vi "DatabaseHand_Element_Get(single).vi"(7 "nd queue":bool, 8 "error in (no error)":errorcluster, 9 "default value":sgl format="%.2f", 10 "name":string, 11 "Database RefNum in":T1) -> (0 "error out":errorcluster, 1 "type":string, 2 "value":sgl format="%.2f", 3 "Database RefNum out":T1, 4 "permissions":string="RW", 5 "group":string, 6 "unit":string)   [LabVIEW 2016]
doc: "This VI finds the RefNum of an existing object with the input Name or creates a new object if the Name is not found or Name is unwired or an empty string.\nCopyright 2001 VI Engineering, Inc."
uses:
  DatabaseHand_RefNum.ctl
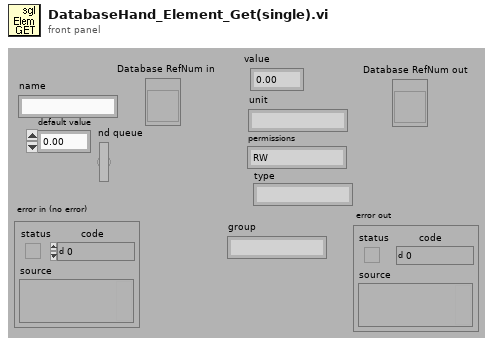
[diagram p1: front panel]
types:
  T1 = typedef "DatabaseHand_RefNum.ctl" = refnum<vi>
  T2 = typedef "DatabaseHand_Element.ctl" = cluster{"name":string, "Database":T3[]}
  T3 = typedef "DatabaseHan_DatabaseElement.ctl" = cluster{"name":string, "value":string, "type":string, "unit":string, "permissions":string, "enqueued":bool, "group":string}
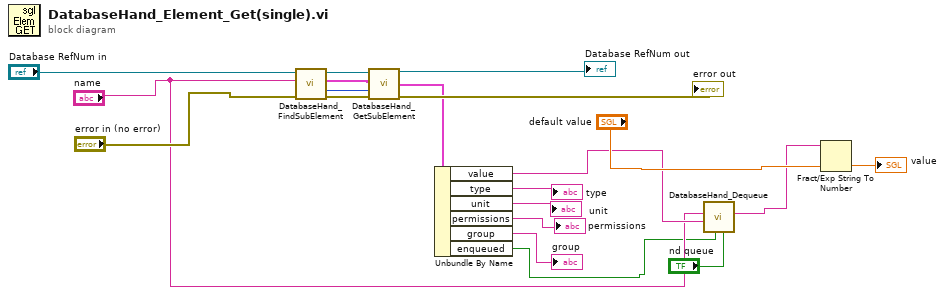
[diagram p0: block diagram]
diagram:
  n1 = call "DatabaseHand_FindSubElement.vi"("error in (no error)"="error in (no error)", "name"="name", "Database RefNum in"="Database RefNum in") -> ("error out"=w16:errorcluster, "index"=w13:i32, "Database"=w17:T2, "Database RefNum out"=w18:T1)  [unwired: 5 out]
  n2 = call "DatabaseHand_GetSubElement.vi"("Database RefNum in"=w18, "Object Data In"=w17, "Index"=w13, "error in (no error)"=w16) -> ("Database RefNum out"=→"Database RefNum out":T1, "Element found"=w12:T3, "error out"=→"error out":errorcluster)  [unwired: 9 out]
  n3 = Unbundle By Name(w12) -> ("value"=w5:string, "type"=→"type":string, "unit"=→"unit":string, "permissions"=→"permissions":string, "group"=→"group":string, "enqueued"=w3:bool)
  n4 = call "DatabaseHand_Dequeue.vi"("non-destructive queue"="nd queue", "queue?"=w3, "value in"=w5, "name"="name") -> ("value out"=w1:string)  [unwired: 1 in, 6 out]
  n5 = Fract/Exp String To Number(string=w1, default (0 dbl)="default value") -> (number=→"value":sgl)  [unwired: 3 out]
